vi "JSONtext and SQlite (requires SQLite LabVIEW).vi"() -> ()   [LabVIEW 2017]
uses:
  <vilib>/drjdpowell/SQLite Library/SQL Statement/SQL Statement.lvclass/SQL Statement.ctl
  <vilib>/drjdpowell/SQLite Library/SQL Connection/Open (path).vi
  <vilib>/drjdpowell/SQLite Library/SQL Statement/Bind UTF-8 Text.vi
  a4ef3bbe-680b-444f-9f5b-3aba932734da.vi
  <vilib>/drjdpowell/SQLite Library/SQL Statement/Bind Integer.vi
  <vilib>/drjdpowell/SQLite Library/SQL Connection/Open (string).vi
  <vilib>/AdvancedString/Path To Command Line String.vi
  <vilib>/drjdpowell/SQLite Library/SQL Connection/Execute SQL (No results).vi
  <vilib>/drjdpowell/SQLite Library/SQL Statement/Error Message.vi
  <vilib>/drjdpowell/SQLite Library/SQL Connection/Execute SQL (Single DBL).vi
  <vilib>/drjdpowell/SQLite Library/SQL Statement/Column UTF-8 Text.vi
  JSON text to Variant.vi
  <vilib>/drjdpowell/SQLite Library/SQL Connection/Connection.lvclass
  JSONtext.lvlib
  <vilib>/drjdpowell/SQLite Library/SQLite.lvlib
  <vilib>/drjdpowell/SQLite Library/SQL Statement/SQL Statement.lvclass
  <vilib>/drjdpowell/SQLite Library/Transaction Helpers/Transaction.lvlib
panel:
  out "Average Age":dbl format="%#.6g"
  out "Returned":cluster{string, dbl, string}[](array[cluster]) caption="Returned people of that age" {"?" format="%#_f"}
  in  "Age":i64=31
  # "This example requires both JSONtext and \"SQLite LabVIEW\" packages"
  # "http://sine.ni.com/nips/cds/view/p/lang/en/nid/212894"
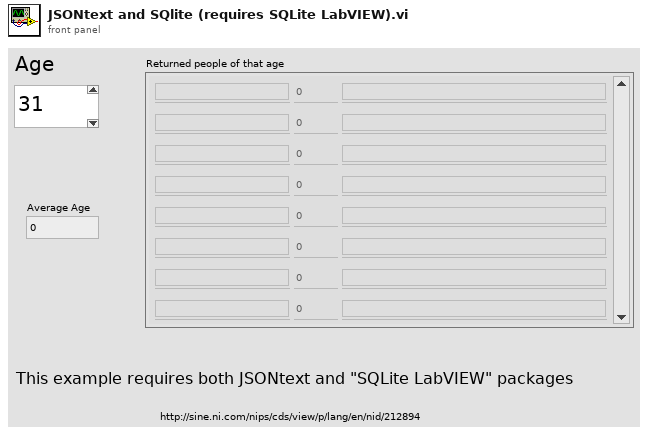
[diagram p1: front panel]
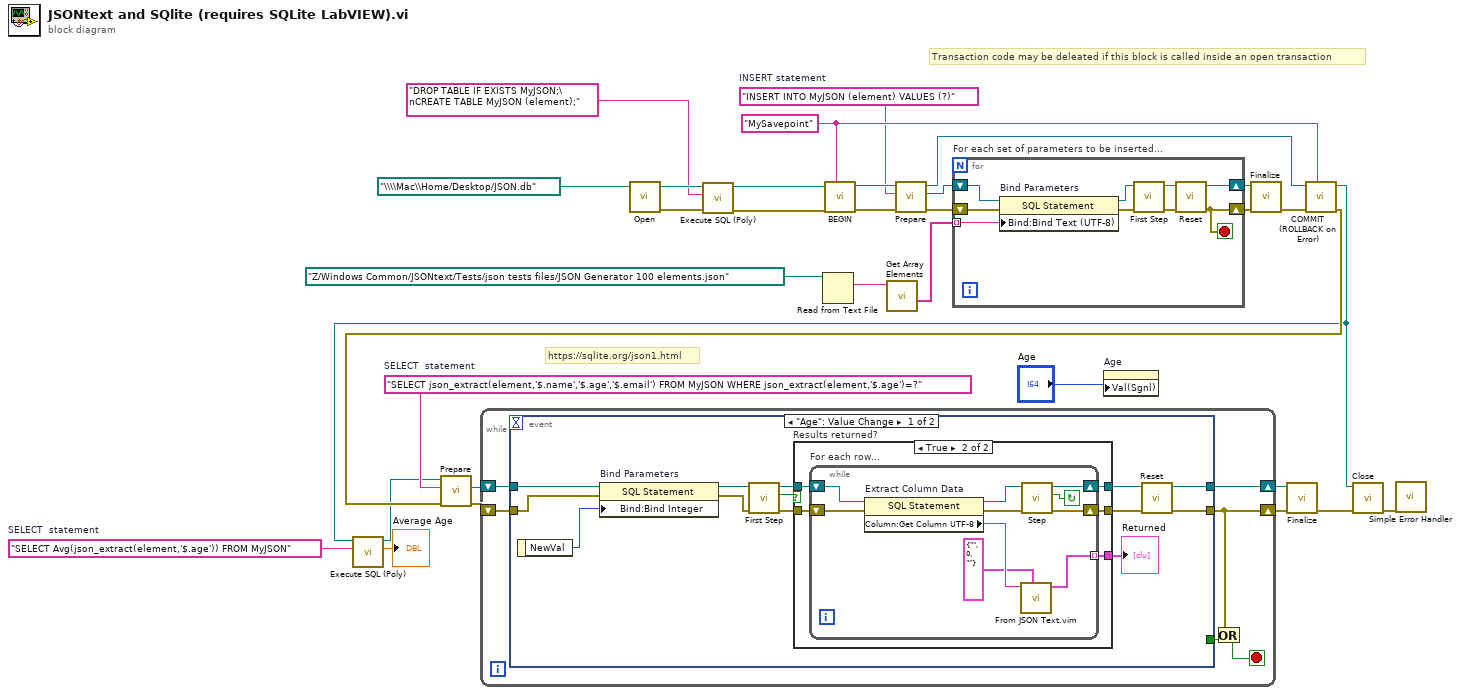
[diagram p0: block diagram]
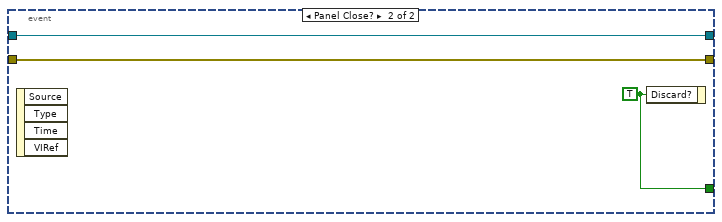
[diagram p3: hidden frame]
diagram:
  w2 = "SELECT Avg(json_extract(element,'$.age')) FROM MyJSON"  # SELECT  statement
  w10 = "SELECT json_extract(element,'$.name','$.age','$.email') FROM MyJSON WHERE json_extract(element,'$.age')=?"  # SELECT  statement
  w25 = "MySavepoint" ("Savepoint name")
  w20 = "INSERT INTO MyJSON (element) VALUES (?)"  # INSERT statement
  # "https://sqlite.org/json1.html"
  # "Transaction code may be deleated if this block is called inside an open transaction"
  n1 = call-poly <vilib>:"Open.vi"("db file"=path "\\\\Mac\\Home/Desktop/JSON.db" ("file (use dialog)")) -> ("error out"=w15:errorcluster, "SQLite Connection out"=w29:refnum<class "Connection.lvclass">)  [unwired: 9 in]
  n2 = call-poly <vilib>:"Execute SQL (Poly).vi"("error in (no error)"=w15, "SQL"="DROP TABLE IF EXISTS MyJSON;\nCREATE TABLE MyJSON (element);", "SQLite Connection in"=w29) -> ("error out"=w14:errorcluster, "SQLite Connection out"=w16:refnum<class "Connection.lvclass">)  [unwired: 7 in]
  n3 = Read from Text File(file (use dialog)=path "Z:/Windows Common/JSONtext/Tests/json tests files/JSON Generator 100 elements.json") -> (text=w31:string)  [unwired: 3 in, 3 out]
  n4 = call <vilib>:"BEGIN.vi"("Savepoint name"=w25, "error in (no error)"=w14, "Connection in"=w16) -> ("error out"=w24:errorcluster, "Connection out"=w23:refnum<class "Connection.lvclass">)  [unwired: 7 in]
  n5 = call "Get Array Elements.vi"("JSON"=w31) -> ("<JSON>"=w17:string[])  [unwired: 8 in, 2 out]
  n6 = call <vilib>:"Prepare.vi"("error in (no error)"=w24, "SQL"=w20, "SQLite Connection in"=w23) -> ("error out"=w19:errorcluster, "SQL Statement out"=w18:refnum<class "SQL Statement.lvclass">, "SQLite Connection out"=w26:refnum<class "Connection.lvclass">)  [unwired: 4 in, 2 out]
  n7 = for "For each set of parameters to be inserted..." {
    shift-right: [w35] -> w21
    shift-left: w18 -> [w41]
    shift-right: [w34] -> w22
    shift-left: w19 -> [w38]
    tunnel: w17 -> [w33] mode=indexing
    stop <- w34 stop-if-true
    n8 = property on="Bind Parameters" class="SQL Statement"(reference=w41, error in=w38, "Bind:Bind Text (UTF-8)"=w33) -> (reference out=w40:refnum<class "SQL Statement.lvclass">, error out=w39:errorcluster)
    n9 = call <vilib>:"First Step.vi"("error in (no error)"=w39, "SQL Statement in"=w40) -> ("error out"=w37:errorcluster, "SQL Statement out"=w36:refnum<class "SQL Statement.lvclass">)  [unwired: 7 in, 1 out]
    n10 = call <vilib>:"Reset.vi"("error in (no error)"=w37, "SQL Statement in"=w36) -> ("error out"=w34:errorcluster, "SQL Statement out"=w35:refnum<class "SQL Statement.lvclass">)  [unwired: 8 in]
  }
  n11 = property on="Age" class="DigNum (strict)"("Val(Sgnl)"="Age") -> ()  [unwired: 2 in, 2 out]
  n12 = call <vilib>:"Finalize.vi"("error in (no error)"=w22, "SQL Statement in"=w21) -> ("error out"=w27:errorcluster)  [unwired: 9 in]
  n13 = call <vilib>:"COMMIT (ROLLBACK on Error).vi"("Savepoint name"=w25, "error in (no error)"=w27, "Connection in"=w26) -> ("error out"=w6:errorcluster, "Connection out"=w3:refnum<class "Connection.lvclass">)  [unwired: 7 in]
  n14 = call-poly <vilib>:"Execute SQL (Poly).vi"("SQL"=w2, "SQLite Connection in"=w3) -> ("Result"=→"Average Age":dbl, "SQLite Connection out"=w4:refnum<class "Connection.lvclass">)  [unwired: 7 in, 1 out]
  n15 = call <vilib>:"Prepare.vi"("error in (no error)"=w6, "SQL"=w10, "SQLite Connection in"=w4) -> ("error out"=w9:errorcluster, "SQL Statement out"=w8:refnum<class "SQL Statement.lvclass">)  [unwired: 4 in, 3 out]
  n16 = while {
    shift-right: [w42] -> w12
    shift-left: w9 -> [w46]
    shift-right: [w47] -> w11
    shift-left: w8 -> [w45]
    stop <- w43 stop-if-true
    n17 = event shown="[0] \"Age\": Value Change" {
      selector: _ -> [_ _]
      dyn-events: _ -> [_ _]
      timeout: _ -> [_ _]
      tunnel: [w50 w78] -> w42
      tunnel: [w49 w79] -> w47
      tunnel: w46 -> [w60 w78]
      tunnel: w45 -> [w57 w79]
      tunnel: [_ w80] -> w44
      event "Age": Value Change {
        n18 = event-data() -> ("NewVal"=w53:i64)  [unwired: 1 in]
        n19 = property on="Bind Parameters" class="SQL Statement"(reference=w57, error in=w60, "Bind:Bind Integer"=w53) -> (reference out=w58:refnum<class "SQL Statement.lvclass">, error out=w59:errorcluster)
        n20 = call <vilib>:"First Step.vi"("error in (no error)"=w59, "SQL Statement in"=w58) -> ("error out"=w55:errorcluster, "Row returned"=w54:bool, "SQL Statement out"=w56:refnum<class "SQL Statement.lvclass">)  [unwired: 7 in]
        n21 = case "Results returned?" shown="True" w54 {
          tunnel: [w62 w67] -> w51
          tunnel: [w61 w66] -> w52
          tunnel: w56 -> [w62 w65]
          tunnel: w55 -> [w61 w64]
          tunnel: [_ w63] -> w48
          frame False {
          }
          frame True {
            n22 = while "For each row..." {
              shift-right: [w76] -> w67
              shift-left: w65 -> [w73]
              shift-right: [w74] -> w66
              shift-left: w64 -> [w72]
              tunnel: [w68] -> w63 mode=indexing
              stop <- w71 continue-if-true
              n23 = property on="Extract Column Data" class="SQL Statement"(reference=w73, error in=w72) -> (reference out=w77:refnum<class "SQL Statement.lvclass">, error out=w75:errorcluster, "Column:Get Column UTF-8"=w70:string)
              n24 = call "From JSON Text.vim"("Data Type and Default Value"=cluster{string, i32, string} {"", 0, ""}, "JSON"=w70) -> ("Variant out"=w68:cluster{string, i32, string})  [unwired: 8 in, 1 out]
              n25 = call <vilib>:"Step.vi"("error in (no error)"=w75, "SQL Statement in"=w77) -> ("error out"=w74:errorcluster, "Row returned"=w71:bool, "SQL Statement out"=w76:refnum<class "SQL Statement.lvclass">)  [unwired: 7 in]
            }
          }
        }
        "Returned" <- w48
        n26 = call <vilib>:"Reset.vi"("error in (no error)"=w52, "SQL Statement in"=w51) -> ("error out"=w50:errorcluster, "SQL Statement out"=w49:refnum<class "SQL Statement.lvclass">)  [unwired: 8 in]
      }
      event Panel Close? {
        w80 = TRUE ("Discard?")
        n27 = event-data() -> ()  [unwired: 1 in, 4 out]
        n28 = event-data("Discard?"=w80) -> ()  [unwired: 1 in, 1 out]
      }
    }
    n29 = Or(x=w42, y=w44) -> (x .or. y?=w43:bool)
  }
  n30 = call <vilib>:"Finalize.vi"("error in (no error)"=w12, "SQL Statement in"=w11) -> ("error out"=w7:errorcluster)  [unwired: 9 in]
  n31 = call-dynamic "Close.vi"("error in (no error)"=w7, "SQLite Connection in"=w3) -> ("error out"=w13:errorcluster)  [unwired: 9 in]
  n32 = call <vilib>:"Simple Error Handler.vi"("error in (no error)"=w13) -> ()  [unwired: 4 in, 5 out]
